vi "AlternatingLEDs.vi"() -> ()   [LabVIEW 2015]
panel:
  out "x = 0?":bool[](array[boolean])
  in  "stop":bool
  out "appended array":bool[](array[boolean])
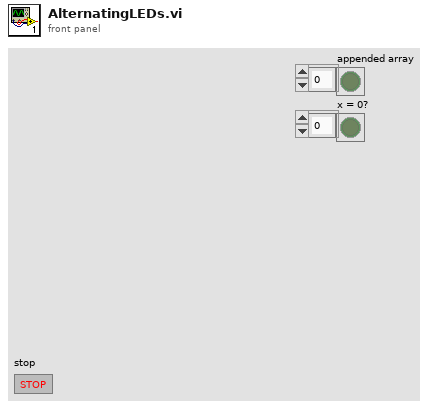
[diagram p1: front panel]
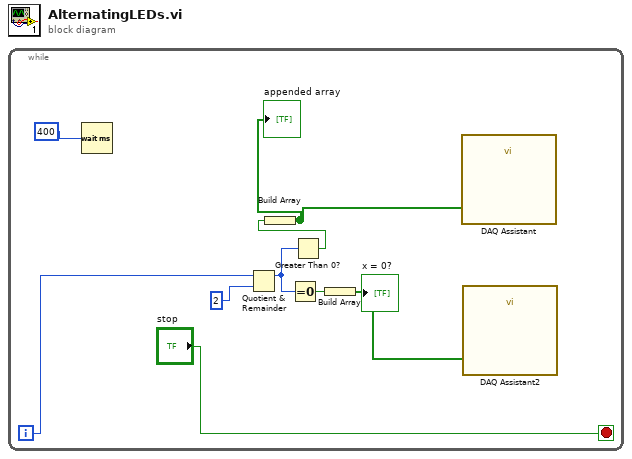
[diagram p0: block diagram]
diagram:
  n1 = while {
    i -> [w7]
    stop <- "stop" stop-if-true
    n2 = Wait (ms)(milliseconds to wait=400) -> ()  [unwired: 1 out]
    n3 = Quotient & Remainder(x=w7, y=2) -> (x-y*floor(x/y)=w3:i32)  [unwired: 1 out]
    n4 = Equal To 0?(x=w3) -> (x = 0?=w5:bool)
    n5 = Greater Than 0?(x=w3) -> (x > 0?=w2:bool)
    n6 = Build Array(w2) -> (w9:bool[])
    "appended array" <- w9
    n7 = Build Array(w5) -> (w4:bool[])
    "x = 0?" <- w4
    n8 = call "DAQ Assistant"("data"=w9) -> ()  [unwired: 17 in, 2 out]
    n9 = call "DAQ Assistant2"("data"=w4) -> ()  [unwired: 17 in, 2 out]
  }
